vi "scan_array_2D.vi"(5 "v1_config":T1={"hardware"=enum."none", "options"="", "repeats"=1, "loops"=1, "VISA"="", "override_VISA"=FALSE} {"loops" min=1; "repeats" min=1}, 7 "v0_config":T1={"hardware"=enum."none", "options"="", "repeats"=1, "loops"=1, "VISA"="", "override_VISA"=FALSE} {"loops" min=1; "repeats" min=1}, 8 "error in":errorcluster, 9 "var mode":enum16{"permutations", "aligned"}(ring), 10 "v1_values":dbl[](array[numeric])=[1.0, 2.0, 3.0, 4.0, 5.0, 6.0, 7.0, 8.0, 9.0, 10.0] format="%#_6p", 11 "v0_values":dbl[](array[numeric])=[1.0, 2.0, 3.0, 4.0, 5.0, 6.0, 7.0, 8.0, 9.0, 10.0] format="%#_6p") -> (0 "error in (no error)":errorcluster={"status"=TRUE, "code"=999, "source"="Failed to align var arrays\nof different length"}, 2 "scan_values":dbl[][](array[numeric]))   [LabVIEW 2017, in "tools.lvlib"]
uses:
  tools.lvlib
  var_config.ctl
  ctrl/var_list.ctl
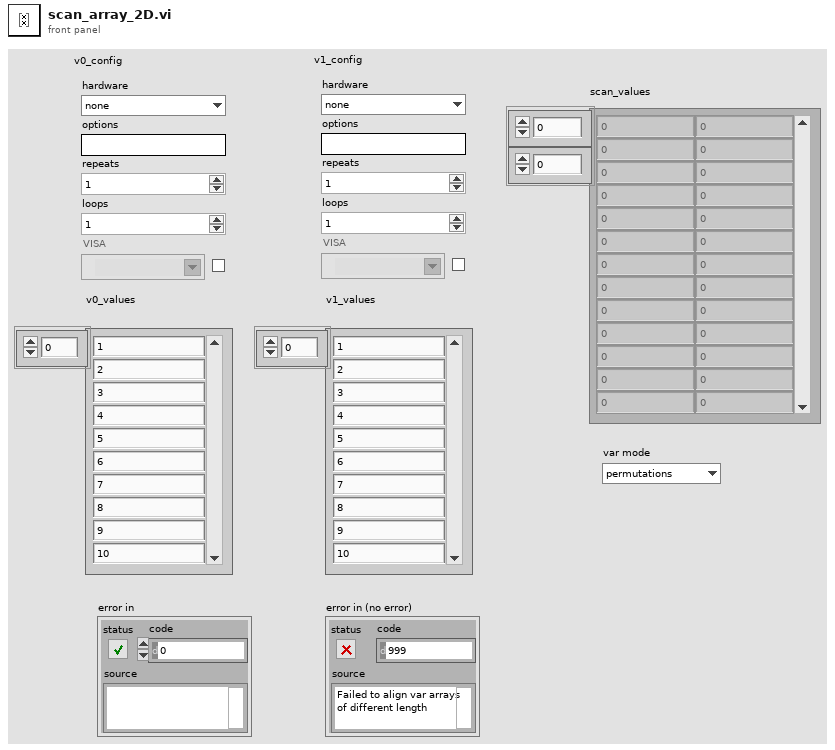
[diagram p1: front panel]
types:
  T1 = typedef "tools.lvlib/var_config.ctl" = cluster{"hardware":T2, "options":string, "repeats":i32, "loops":i32, "VISA":refnum<visa-resource-name>, "override_VISA":bool}
  T2 = typedef "var_list.ctl" = enum16{"none", "AO voltage (V)", "delay (s)", "generic", "microwaves (GHz)", "radiant (nm)", "radiant thg (nm)", "sirah (nm)", "sirah_shg (nm)", "tenma voltage (V)", "wait (s)", "wf_freq (Hz)", "wf_amp (V)", "wf_amp_multi (V)", "wf_offset (V)", "wf_low_level (V)", "wf_high_level (V)", "wf_period (s)", "wf_pulse_width (s)", "wf_sample_rate (Sa/s)", "wf_multi_amp", "wf_multi_freq", "wf_arb_4chan", "WS7 setpoint (nm)"}
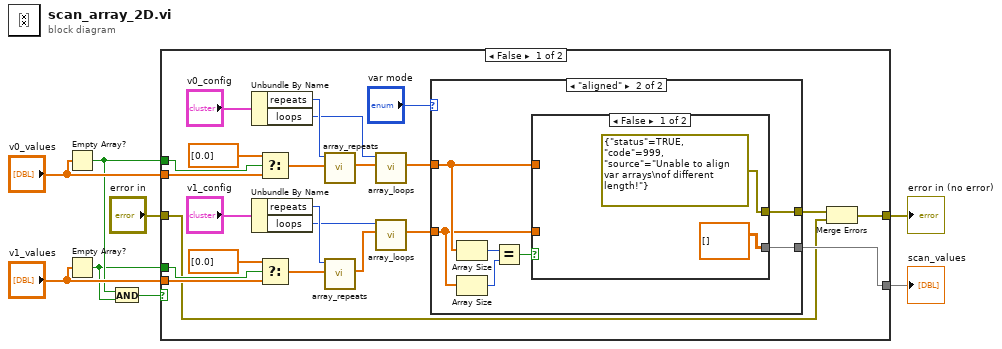
[diagram p0: block diagram]
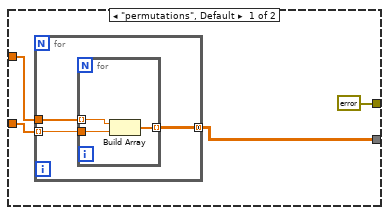
[diagram p2: hidden frame]
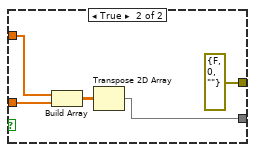
[diagram p3: hidden frame]
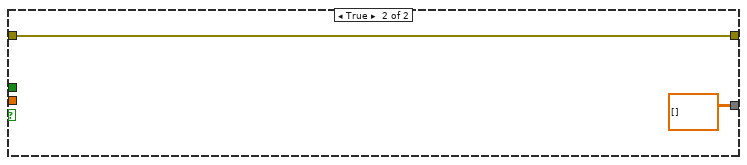
[diagram p4: hidden frame]
diagram:
  n1 = Empty Array?(array="v0_values") -> (empty?=w5:bool)
  n2 = Empty Array?(array="v1_values") -> (empty?=w4:bool)
  n3 = And(x=w5, y=w4) -> (x .and. y?=w1:bool)
  n4 = case shown="False" w1 {
    tunnel: [w20 w57] -> w8
    tunnel: "v1_values" -> [w17 _]
    tunnel: "v0_values" -> [w15 _]
    tunnel: w5 -> [w12 _]
    tunnel: w4 -> [w11 _]
    tunnel: [w10 dbl[][] []] -> w3
    tunnel: "error in" -> [w9 w57]
    frame False {
      n5 = Unbundle By Name("v0_config") -> ("repeats"=w28:i32, "loops"=w26:i32)
      n6 = Unbundle By Name("v1_config") -> ("repeats"=w30:i32, "loops"=w22:i32)
      n7 = Select(t=dbl[] [0.0], s=w12, f=w15) -> (s? t:f=w14:dbl[])
      n8 = Select(t=dbl[] [0.0], s=w11, f=w17) -> (s? t:f=w16:dbl[])
      n9 = call "array_repeats.vi"("values_IN"=w14, "repeats"=w28) -> ("values_OUT"=w27:dbl[])  [unwired: 9 in]
      n10 = call "array_repeats.vi"("values_IN"=w16, "repeats"=w30) -> ("values_OUT"=w24:dbl[])  [unwired: 9 in]
      n11 = call "array_loops.vi"("values_IN"=w27, "loops"=w26) -> ("values_OUT"=w25:dbl[])  [unwired: 9 in]
      n12 = call "array_loops.vi"("values_IN"=w24, "loops"=w22) -> ("values_OUT"=w23:dbl[])  [unwired: 9 in]
      n13 = case shown="\"aligned\"" "var mode" {
        tunnel: [w35 w45] -> w10
        tunnel: w25 -> [w34 w44]
        tunnel: w23 -> [w33 w43]
        tunnel: [errorcluster {"status"=FALSE, "code"=0, "source"=""} ("error in (no error)") w42] -> w19
        frame "permutations", Default {
          n14 = for {
            tunnel: w34 -> [w38]
            tunnel: w33 -> [w37] mode=indexing
            tunnel: [w36] -> w35 mode=concatenating
            n15 = for {
              tunnel: w38 -> [w41] mode=indexing
              tunnel: w37 -> [w40]
              tunnel: [w39] -> w36 mode=indexing
              n16 = Build Array(w41, w40) -> (w39:dbl[])
            }
          }
        }
        frame "aligned" {
          n17 = Array Size(array=w44) -> (size(s)=w48:i32)
          n18 = Array Size(array=w43) -> (size(s)=w47:i32)
          n19 = Equal?(x=w48, y=w47) -> (x = y?=w46:bool)
          n20 = case shown="False" w46 {
            tunnel: [dbl[][] [] w52] -> w45
            tunnel: w44 -> [_ w55]
            tunnel: w43 -> [_ w54]
            tunnel: [errorcluster {"status"=TRUE, "code"=999, "source"="Unable to align var arrays\nof different length!"} ("error in (no error)") errorcluster {"status"=FALSE, "code"=0, "source"=""} ("error in (no error)")] -> w42
            frame False {
            }
            frame True {
              n21 = Build Array(w55, w54) -> (w53:dbl[][])
              n22 = Transpose 2D Array(2D array=w53) -> (transposed array=w52:dbl[][])
            }
          }
        }
      }
      n23 = Merge Errors(w19, w9) -> (w20:errorcluster)
    }
    frame True {
    }
  }
  "error in (no error)" <- w8
  "scan_values" <- w3
